vi "real_time_trace_avg.vi"(1 "C1 enabled":bool=TRUE caption="Enabled?", 3 "C2 enabled":bool=TRUE caption="Enabled?", 7 "scope Q data":T1) -> (4 "Channel 1 RT avg":waveform(dbl)(graph), 13 "Error out":errorcluster, 15 "Channel 2 RT avg":waveform(dbl)(graph))   [LabVIEW 2023]
uses:
  <vilib>/Waveform/WDTOps.llb/WDT Align Waveform Timestamps DBL.vi
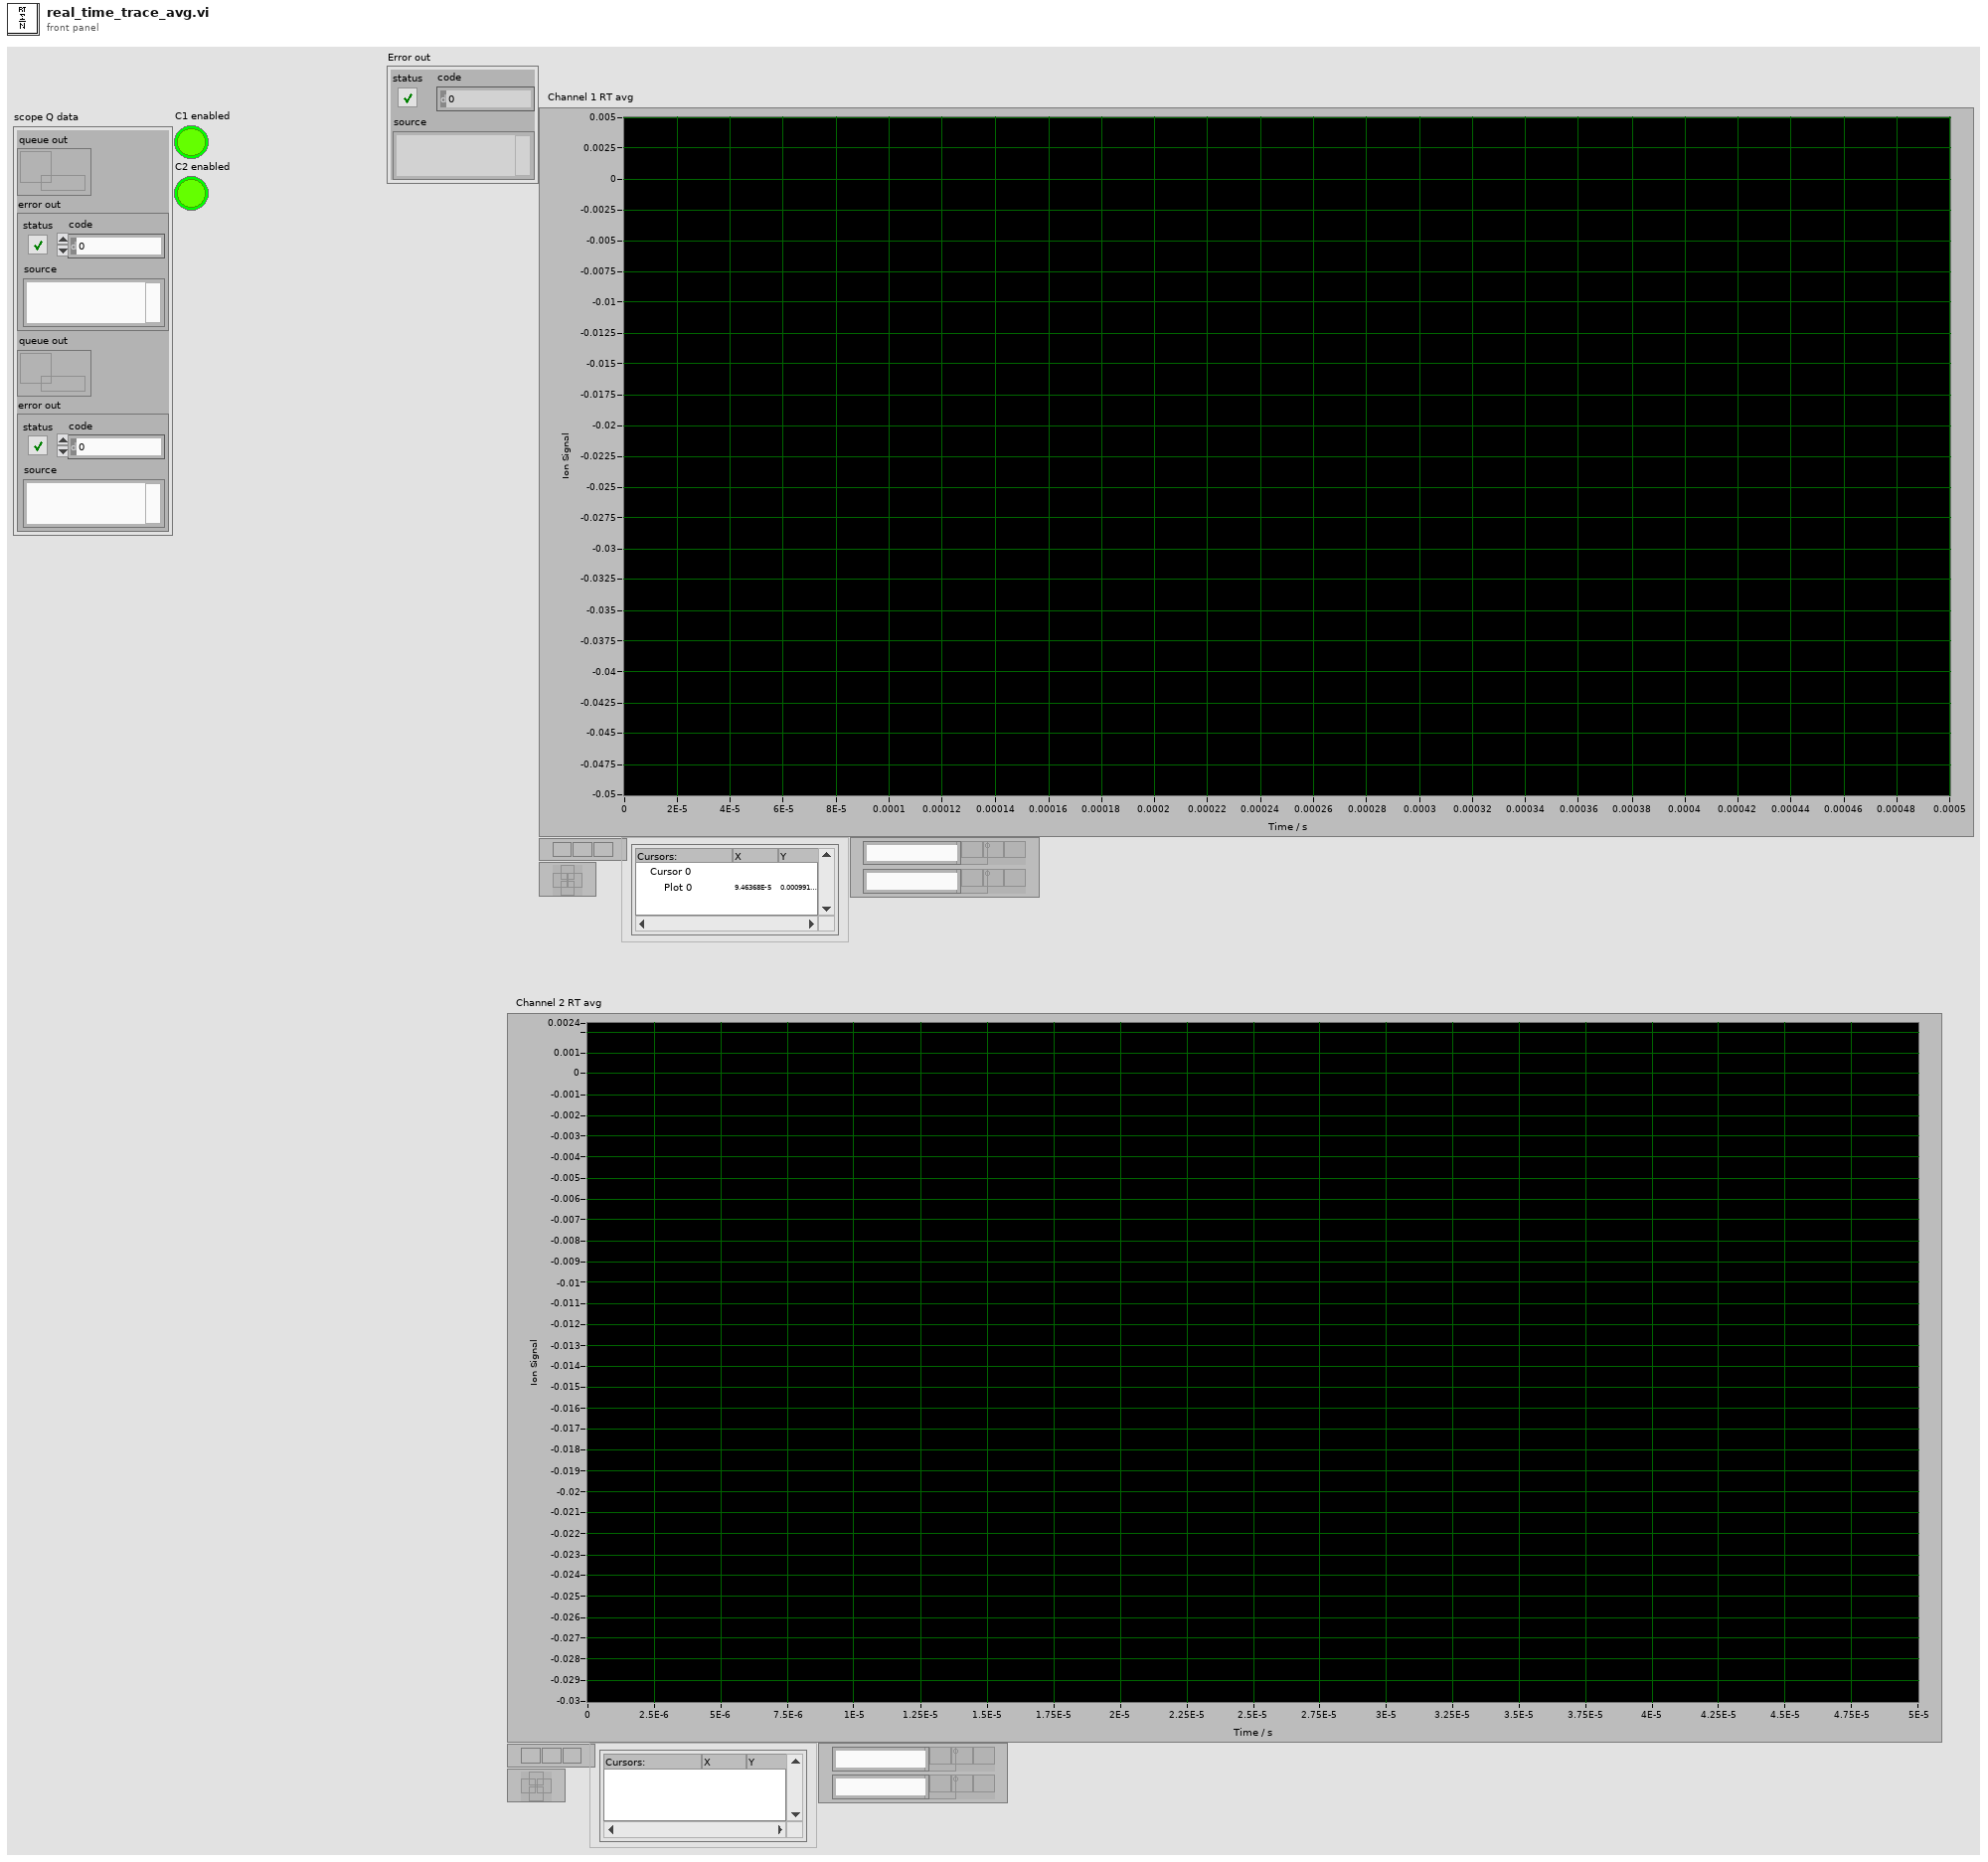
[diagram p1: front panel]
types:
  T1 = cluster{"queue out":refnum<queue>, "error out":errorcluster, "queue out":refnum<queue>, "error out":errorcluster}
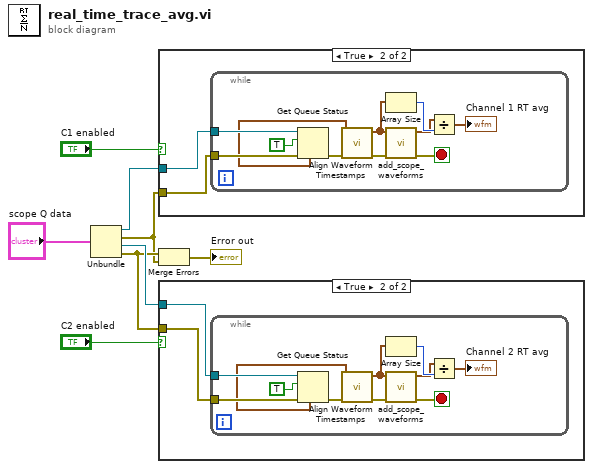
[diagram p0: block diagram]
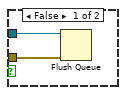
[diagram p2: hidden frame]
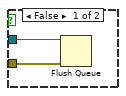
[diagram p3: hidden frame]
diagram:
  n1 = Unbundle("scope Q data") -> ("queue out"=w7:refnum<queue>, "error out"=w2:errorcluster, "queue out"=w5:refnum<queue>, "error out"=w3:errorcluster)
  n2 = case shown="True" "C1 enabled" {
    tunnel: w7 -> [w10 w12]
    tunnel: w2 -> [w9 w11]
    frame False {
      n3 = Flush Queue(queue=w10, error in (no error)=w9) -> ()  [unwired: 3 out]
    }
    frame True {
      n4 = while {
        tunnel: w12 -> [w23]
        tunnel: w11 -> [w22]
        stop <- w14 stop-if-true
        n5 = Get Queue Status(queue=w23, return elements? (F)=TRUE, error in (no error)=w22) -> (error out=w21:errorcluster, elements=w19:waveform(dbl)[])  [unwired: 6 out]
        n6 = call-poly <vilib>:"Align Waveform Timestamps.vi"("error in (no error)"=w21, "waveforms in"=w19) -> ("error out"=w18:errorcluster, "waveforms out"=w16:waveform(dbl)[])  [unwired: 8 in]
        n7 = Array Size(array=w16) -> (size(s)=w17:i32)
        n8 = call "add_scope_waveforms.vi"("Error in (no error)"=w18, "Waveform array"=w16) -> ("Error out"=w14:errorcluster, "Summed waveform"=w15:waveform(dbl))  [unwired: 8 in]
        n9 = Divide(x=w15, y=w17) -> (x/y=→"Channel 1 RT avg":waveform(dbl))
      }
    }
  }
  n10 = Merge Errors(w3, w2) -> (→"Error out":errorcluster)
  n11 = case shown="True" "C2 enabled" {
    tunnel: w5 -> [w25 w27]
    tunnel: w3 -> [w24 w26]
    frame False {
      n12 = Flush Queue(queue=w25, error in (no error)=w24) -> ()  [unwired: 3 out]
    }
    frame True {
      n13 = while {
        tunnel: w27 -> [w38]
        tunnel: w26 -> [w37]
        stop <- w29 stop-if-true
        n14 = Get Queue Status(queue=w38, return elements? (F)=TRUE, error in (no error)=w37) -> (error out=w36:errorcluster, elements=w34:waveform(dbl)[])  [unwired: 6 out]
        n15 = call-poly <vilib>:"Align Waveform Timestamps.vi"("error in (no error)"=w36, "waveforms in"=w34) -> ("error out"=w33:errorcluster, "waveforms out"=w31:waveform(dbl)[])  [unwired: 8 in]
        n16 = Array Size(array=w31) -> (size(s)=w32:i32)
        n17 = call "add_scope_waveforms.vi"("Error in (no error)"=w33, "Waveform array"=w31) -> ("Error out"=w29:errorcluster, "Summed waveform"=w30:waveform(dbl))  [unwired: 8 in]
        n18 = Divide(x=w30, y=w32) -> (x/y=→"Channel 2 RT avg":waveform(dbl))
      }
    }
  }
